vi "UI Status Change.vi"(8 "error in (no error)":errorcluster, 10 "Status":string, 11 "Chat Room Model in":refnum<class "Chat Window Model.lvclass">) -> (0 "error out":errorcluster, 3 "Chat Room Model out":refnum<class "Chat Window Model.lvclass">)   [LabVIEW 2020, in "Chat Window Model.lvlib" / "Chat Window Model.lvclass"]
uses:
  Chat Window Model.lvclass
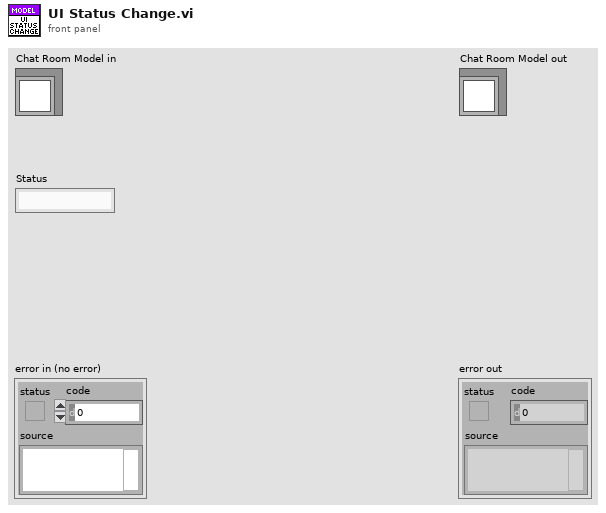
[diagram p1: front panel]
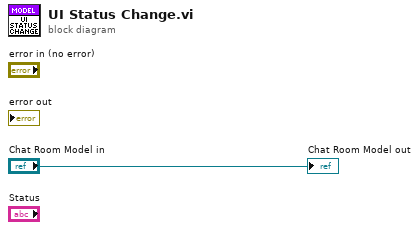
[diagram p0: block diagram]
diagram:
  "Chat Room Model out" <- "Chat Room Model in"
